vi "EditValue.vi"(8 "error in (no error)":errorcluster, 10 "Bounds":T1, 11 "Double D Element.lvclass":refnum<class "Double D Element.lvclass">) -> (0 "error out":errorcluster, 1 "Tabbed out?":bool, 2 "Value changed?":bool, 3 "Double D Element.lvclass":refnum<class "Double D Element.lvclass">)   [LabVIEW 2018, in "D Datagrid Library.lvlib" / "Double D Element.lvclass"]
uses:
  Double D Element.lvclass
  <vilib>/Utility/miscctls.llb/LVRectTypeDef.ctl
panel:
  in  "Value":dbl
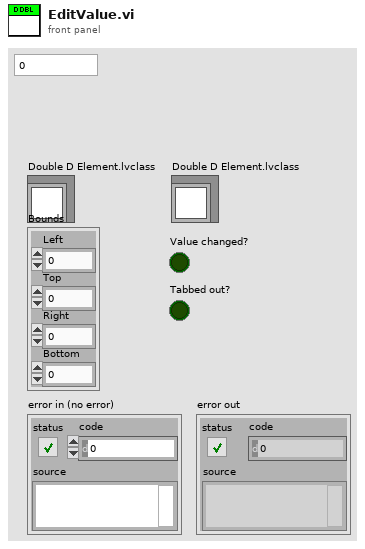
[diagram p1: front panel]
types:
  T1 = typedef "LVRectTypeDef.ctl" = cluster{"Left":i16, "Top":i16, "Right":i16, "Bottom":i16}
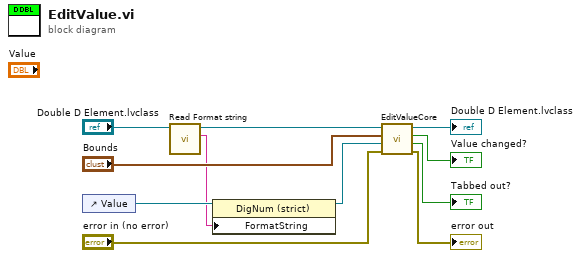
[diagram p0: block diagram]
diagram:
  n1 = control-ref of="Value"() -> (w3:refnum<vi>)
  n2 = call-dynamic "Read Format string.vi"("Double D Element in"="Double D Element.lvclass") -> ("Format string"=w2:string, "Double D Element out"=w4:refnum<class "Double D Element.lvclass">)  [unwired: 8 in, 1 out]
  n3 = property class="DigNum (strict)"(reference=w3, "FormatString"=w2) -> (reference out=w1:refnum<vi>)  [unwired: 1 in, 1 out]
  n4 = call-dynamic "EditValueCore.vi"("error in (no error)"="error in (no error)", "Value field reference"=w1, "Bounds"="Bounds", "DatagridElement in"=w4) -> ("error out"=→"error out":errorcluster, "Tabbed out?"=→"Tabbed out?":bool, "Value changed?"=→"Value changed?":bool, "DatagridElement out"=→"Double D Element.lvclass":refnum<class "Double D Element.lvclass">)  [unwired: 4 in]
